vi "Lift_off.vi"() -> ()   [LabVIEW 2012]
uses:
  Global 2.vi
panel:
  in  "Normalization":bool=TRUE
  in  "Fs":dbl[](array[numeric])
  in  "Update data":bool
  in  "Filter":bool=TRUE
  out "Pulse signal in graph dV":dbl[][](graph)
  in  "low cutoff freq: fl":dbl=40.0 format="%0.2f"
  out "Pulse signal in graph d2V":dbl[][](graph)
  out "Pulse signal in graph":dbl[][](graph)
  in  "stop":bool
  in  "Open":bool
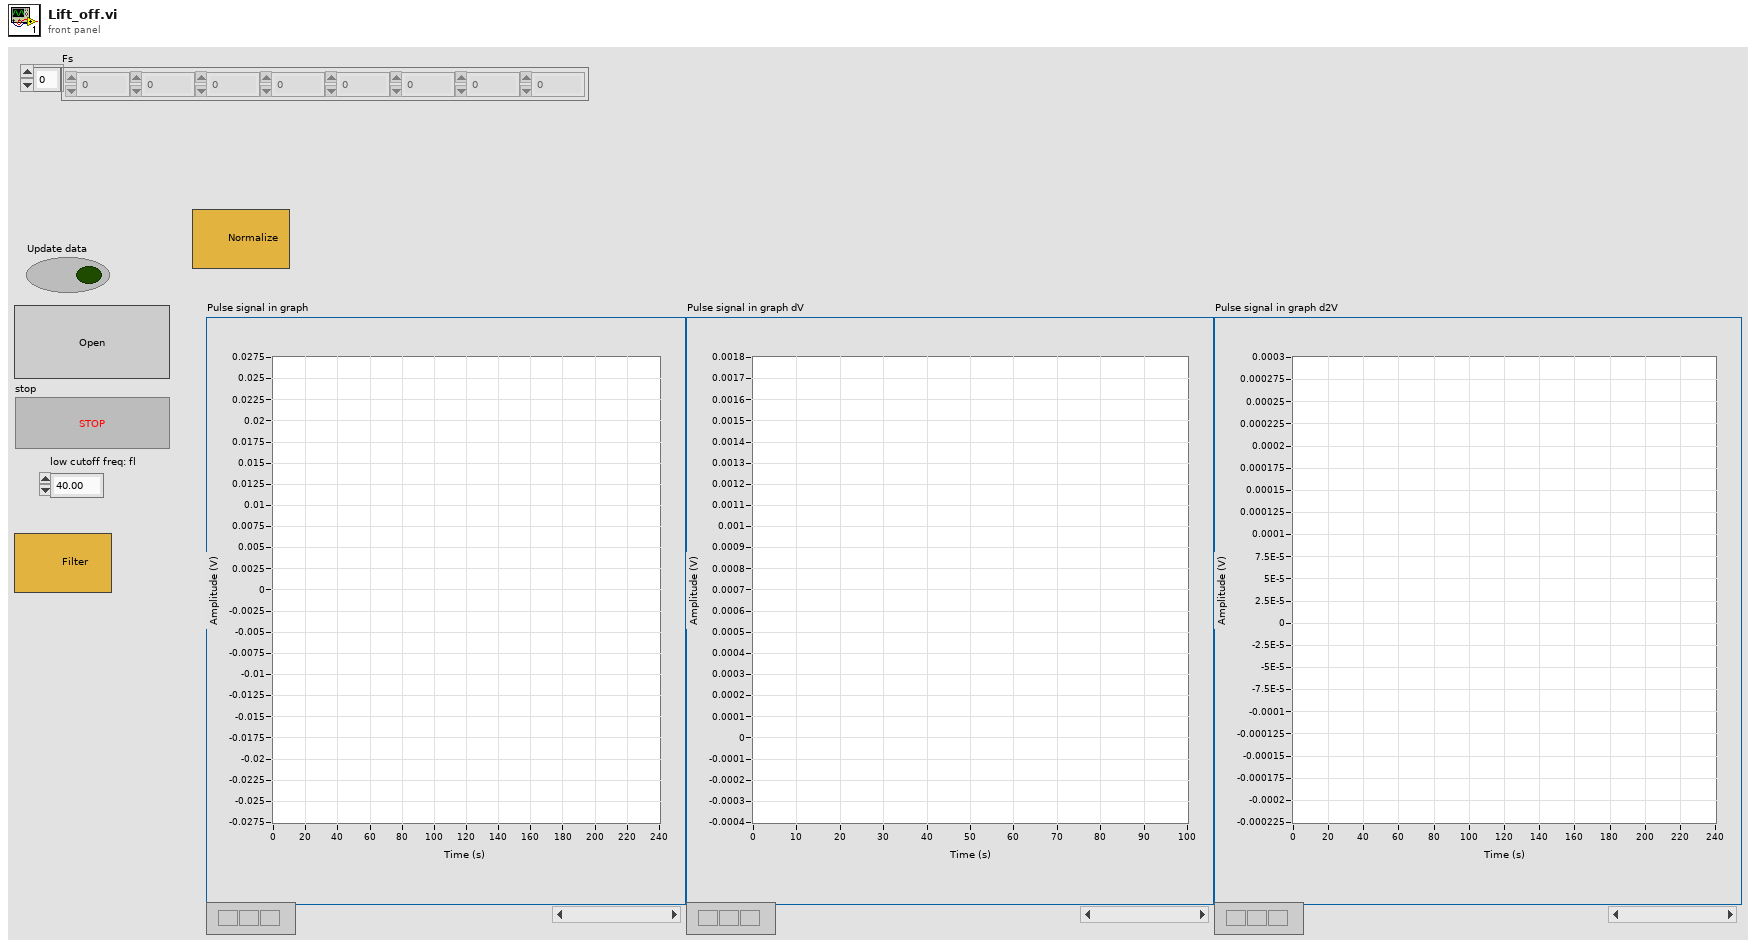
[diagram p1: front panel]
types:
  T1 = cluster{"low cutoff freq: fl":dbl, dbl[], "Signal out":dbl[]}
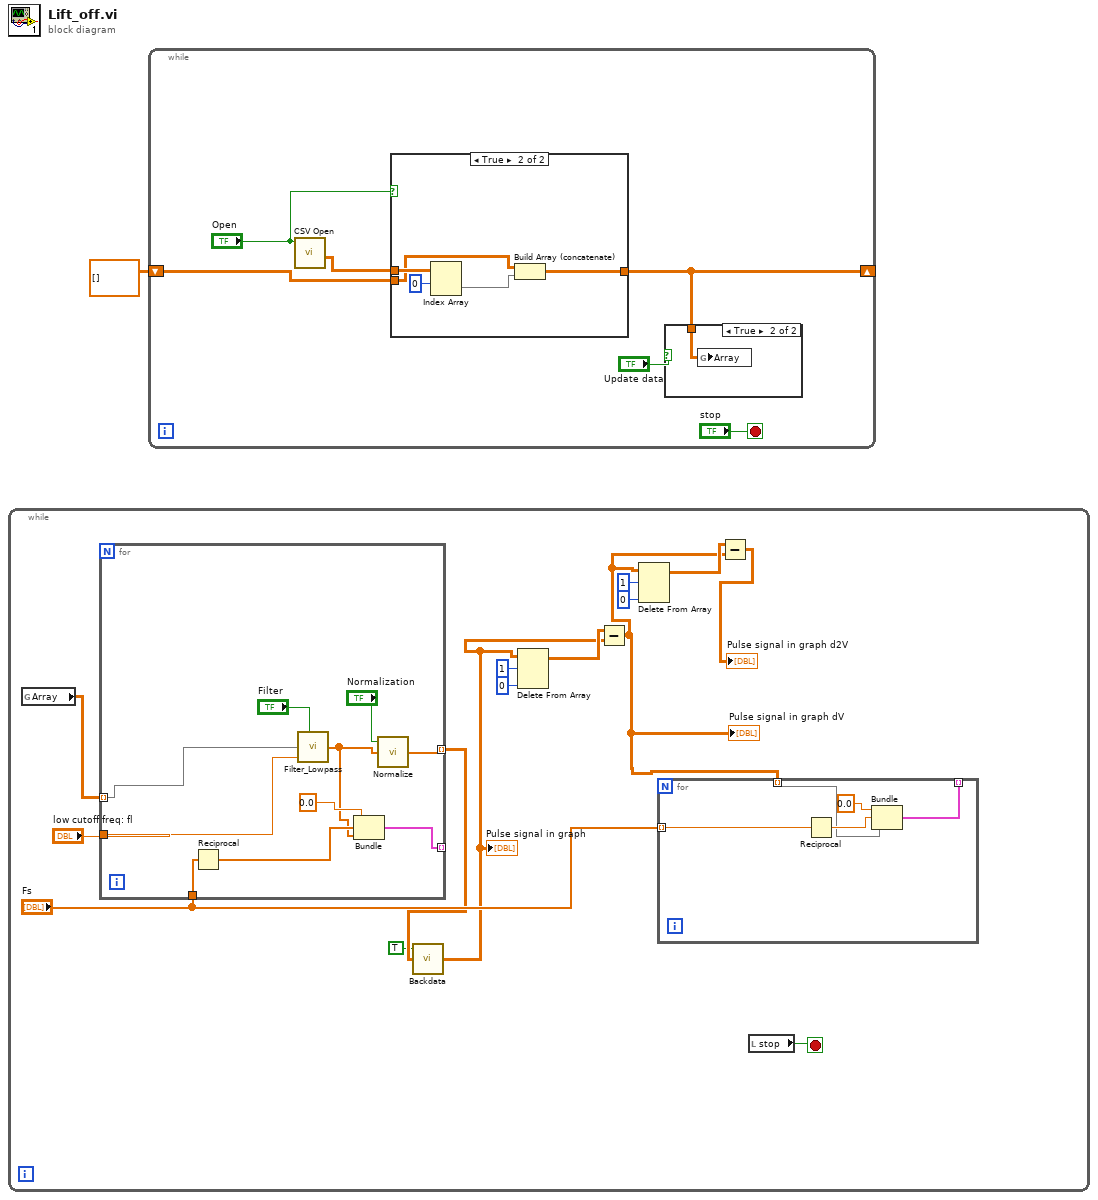
[diagram p0: block diagram]
diagram:
  n1 = while {
    stop <- w12 stop-if-true
    n2 = global read "Global 2.vi" "Array"() -> (w7:dbl[][])
    n3 = for {
      tunnel: w7 -> [w29] mode=indexing
      tunnel: [w23] -> w4 mode=indexing
      tunnel: "low cutoff freq: fl" -> [w31]
      tunnel: "Fs" -> [w26]
      tunnel: [w25] -> _ mode=indexing
      n4 = Reciprocal(x=w26) -> (1/x=w27:dbl[])
      n5 = call "Filter_Lowpass.vi"("Filter"="Filter", "Pulse signal in"=w29, "low cutoff freq: fl"=w31) -> ("Signal out"=w24:dbl[])  [unwired: 6 in]
      n6 = Bundle("low cutoff freq: fl"=0.0, w27, "Signal out"=w24) -> (w25:T1)  [unwired: 1 in]
      n7 = call "Normalize.vi"("Normalization"="Normalization", "Pulse signal in"=w24) -> ("Pulse signal out"=w23:dbl[])  [unwired: 5 in]
    }
    n8 = call "Backdata.vi"("Array in"=w4, "Backdata"=TRUE) -> ("Array out"=w3:dbl[][])  [unwired: 1 in]
    "Pulse signal in graph" <- w3
    n9 = Delete From Array(array=w3, length=1, index (col)=0 ("disabled index (col)")) -> (array with subset deleted=w13:dbl[][])  [unwired: 1 in, 1 out]
    n10 = Subtract(x=w13, y=w3) -> (x-y=w5:dbl[][])
    "Pulse signal in graph dV" <- w5
    n11 = Delete From Array(array=w5, length=1, index (col)=0 ("disabled index (col)")) -> (array with subset deleted=w11:dbl[][])  [unwired: 1 in, 1 out]
    n12 = for {
      tunnel: [w18] -> _ mode=indexing
      tunnel: w5 -> [w19] mode=indexing
      tunnel: "Fs" -> [w17] mode=indexing
      n13 = Reciprocal(x=w17) -> (1/x=w20:dbl)
      n14 = Bundle("low cutoff freq: fl"=0.0, w20, w19) -> (w18:cluster{"low cutoff freq: fl":dbl, dbl, dbl[]})  [unwired: 1 in]
    }
    n15 = Subtract(x=w11, y=w5) -> (x-y=→"Pulse signal in graph d2V":dbl[][])
    n16 = local read "stop"() -> (w12:bool)
  }
  n17 = while {
    shift-right: [w33] -> _
    shift-left: dbl[][] [] -> [w36]
    stop <- "stop" stop-if-true
    n18 = call "CSV Open.vi"("Open"="Open") -> ("2D Array Out"=w37:dbl[][])  [unwired: 10 in]
    n19 = case shown="True" "Open" {
      tunnel: w37 -> [_ w44]
      tunnel: [w39 w41] -> w33
      tunnel: w36 -> [w39 w40]
      frame False {
      }
      frame True {
        n20 = Index Array(array=w44, index (row)=0) -> (element=w42:dbl[])  [unwired: 1 in]
        n21 = Build Array (concatenate)(w40, w42) -> (w41:dbl[][])
      }
    }
    n22 = case shown="True" "Update data" {
      tunnel: w33 -> [_ w38]
      frame False {
      }
      frame True {
        n23 = global write "Global 2.vi" "Array"(w38) -> ()
      }
    }
  }
